vi "readInEthernetXml.vi"(8 "error in (no error)":errorcluster, 10 "xml in":refnum<class "NativeXML.lvclass">, 11 "deviceDataBase in":refnum<class "deviceDataBase.lvclass">) -> (0 "error out":errorcluster, 1 "device.lvclass out":refnum<class "device.lvclass">, 3 "deviceDataBase out":refnum<class "deviceDataBase.lvclass">)   [LabVIEW 2011, in "Tools.lvlib" / "DatabaseHelpers.lvlib" / "deviceDataBase.lvclass"]
uses:
  deviceDataBase.lvclass
  Database Objects/device/device.lvclass
  NativeXML/NativeXML.lvclass
  Database Objects/device/EthernetSupply/ethernetSupply.lvclass
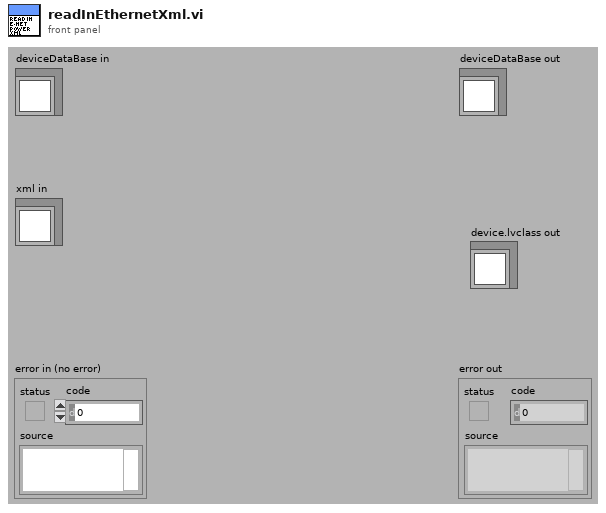
[diagram p1: front panel]
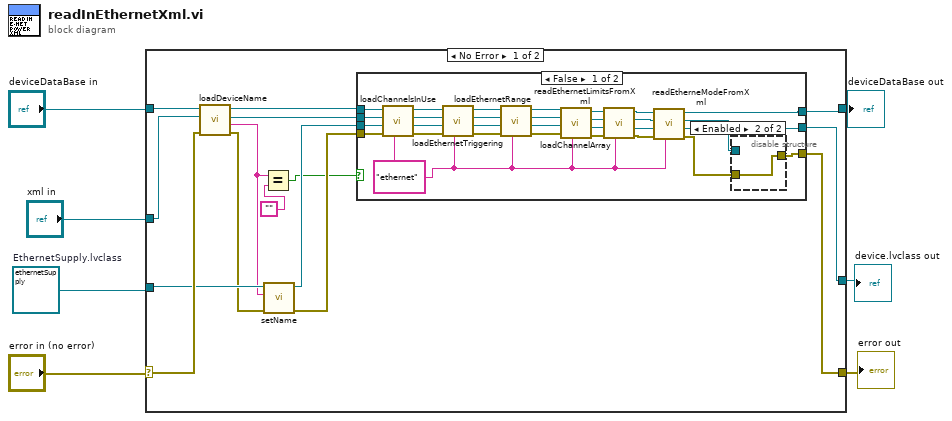
[diagram p0: block diagram]
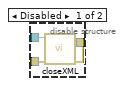
[diagram p2: hidden frame]
diagram:
  w1 = refnum<class "ethernetSupply.lvclass"> refnum  # EthernetSupply.lvclass
  n1 = case shown="No Error" "error in (no error)" {
    selector: "error in (no error)" -> [w21 w61]
    tunnel: [w8 w61] -> w5
    tunnel: [w12 w60] -> w4
    tunnel: "deviceDataBase in" -> [w22 w60]
    tunnel: "xml in" -> [w20 _]
    tunnel: w1 -> [w19 _]
    tunnel: [w13 _] -> w3
    frame No Error {
      n2 = call "loadDeviceName.vi"("error in (no error)"=w21, "NativeXML in"=w20, "deviceDataBase in"=w22) -> ("error out"=w18:errorcluster, "deviceName"=w9:string, "NativeXML out"=w15:refnum<class "NativeXML.lvclass">, "deviceDataBase out"=w17:refnum<class "deviceDataBase.lvclass">)  [unwired: 5 in]
      n3 = Equal?(x=w9, y="") -> (x = y?=w11:bool)
      n4 = call "setName.vi"("error in (no error)"=w18, "name"=w9, "device.lvclass in"=w19) -> ("error out"=w16:errorcluster, "device.lvclass out"=w14:refnum<class "ethernetSupply.lvclass">)  [unwired: 7 in]
      n5 = case shown="False" w11 {
        tunnel: w17 -> [w52 w59]
        tunnel: w16 -> [w51 w57]
        tunnel: w15 -> [w50 _]
        tunnel: w14 -> [w49 w58]
        tunnel: [w32 w57] -> w8
        tunnel: [w24 w58] -> w13
        tunnel: [w25 w59] -> w12
        frame False {
          w29 = "ethernet"
          n6 = call "loadChannelsInUse.vi"("type"=w29, "error in (no error)"=w51, "device.lvclass"=w49, "NativeXML in"=w50, "deviceDataBase in"=w52) -> ("error out"=w45:errorcluster, "device.lvclass out"=w46:refnum<class "device.lvclass">, "NativeXML out"=w47:refnum<class "NativeXML.lvclass">, "deviceDataBase out"=w48:refnum<class "deviceDataBase.lvclass">)  [unwired: 3 in]
          n7 = call "loadEthernetTriggering.vi"("type"=w29, "error in (no error)"=w45, "device.lvclass"=w46, "xml in"=w47, "deviceDataBase in"=w48) -> ("error out"=w39:errorcluster, "device.lvclass out"=w38:refnum<class "device.lvclass">, "xml out"=w37:refnum<class "NativeXML.lvclass">, "deviceDataBase out"=w44:refnum<class "deviceDataBase.lvclass">)  [unwired: 3 in]
          n8 = call "loadEthernetRange.vi"("type"=w29, "error in (no error)"=w39, "device.lvclass"=w38, "xml in"=w37, "deviceDataBase in"=w44) -> ("error out"=w40:errorcluster, "device.lvclass out"=w41:refnum<class "device.lvclass">, "xml out"=w42:refnum<class "NativeXML.lvclass">, "deviceDataBase out"=w43:refnum<class "deviceDataBase.lvclass">)  [unwired: 3 in]
          n9 = call "loadChannelArray.vi"("type"=w29, "error in (no error)"=w40, "device.lvclass"=w41, "NativeXML in"=w42, "deviceDataBase in"=w43) -> ("error out"=w35:errorcluster, "device.lvclass out"=w34:refnum<class "device.lvclass">, "NativeXML out"=w33:refnum<class "NativeXML.lvclass">, "deviceDataBase out"=w36:refnum<class "deviceDataBase.lvclass">)  [unwired: 3 in]
          n10 = call "readEthernetLimitsFromXml.vi"("type"=w29, "error in (no error)"=w35, "device.lvclass"=w34, "xml in"=w33, "deviceDataBase in"=w36) -> ("error out"=w31:errorcluster, "device.lvclass out"=w26:refnum<class "device.lvclass">, "xml out"=w27:refnum<class "NativeXML.lvclass">, "deviceDataBase out"=w28:refnum<class "deviceDataBase.lvclass">)  [unwired: 3 in]
          n11 = call "readEtherneModeFromXml.vi"("type"=w29, "error in (no error)"=w31, "device.lvclass"=w26, "xml in"=w27, "deviceDataBase in"=w28) -> ("error out"=w30:errorcluster, "device.lvclass out"=w24:refnum<class "device.lvclass">, "xml out"=w23:refnum<class "NativeXML.lvclass">, "deviceDataBase out"=w25:refnum<class "deviceDataBase.lvclass">)  [unwired: 3 in]
          n12 = disable-structure shown="Enabled" {
            disable-tunnel: w23 -> [w55 _]
            disable-tunnel: w30 -> [w54 w56]
            disable-tunnel: [w53 w56] -> w32
            frame Disabled {
              n13 = call "closeXML.vi"("error in (no error)"=w54, "NativeXML in"=w55) -> ("error out"=w53:errorcluster)  [unwired: 9 in]
            }
            frame Enabled {
            }
          }
        }
        frame True {
        }
      }
    }
    frame Error {
    }
  }
  "error out" <- w5
  "deviceDataBase out" <- w4
  "device.lvclass out" <- w3
